vi "InGen.vi"() -> (0 "Variables de planta":u16[](array[numeric]))   [LabVIEW 2017, in "Lib_Esclavo_Ingen.lvlib"]
doc: "Simulador de variables eléctricas. Planta InGEN INC."
uses:
  <vilib>/Analysis/baseanly.llb/Mean (DBL).vi
  Lib_Esclavo_Ingen.lvlib
  <vilib>/Analysis/NI_AALBase.lvlib
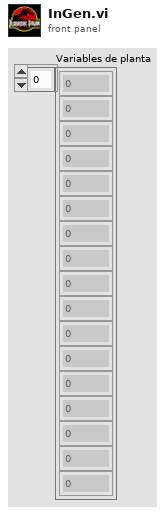
[diagram p1: front panel]
types:
  T1 = enum16{"Tensiones", "Corrientes", "Potencias", "Factores de Potencia", "Frecuencia"}
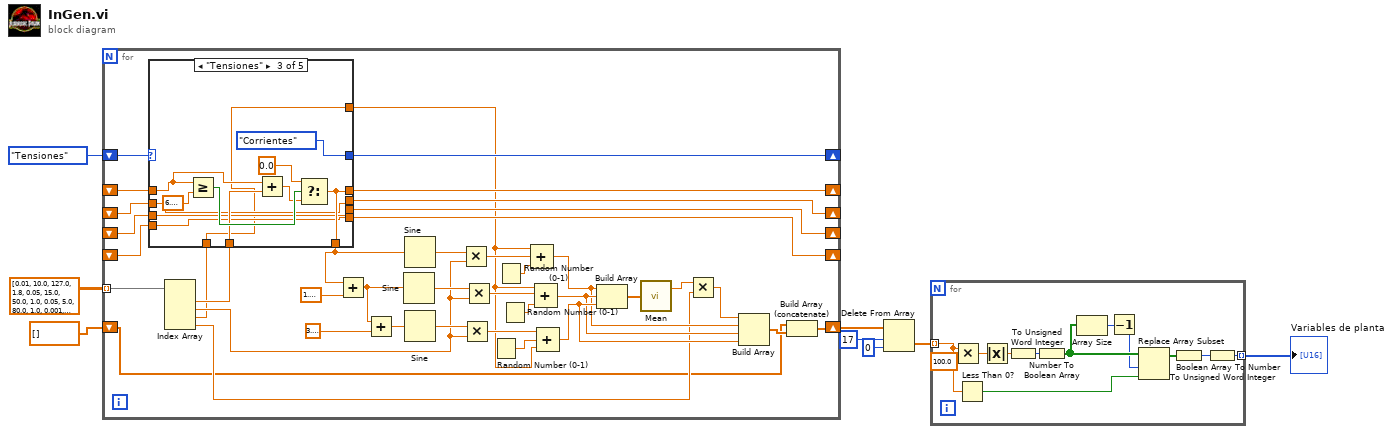
[diagram p0: block diagram]
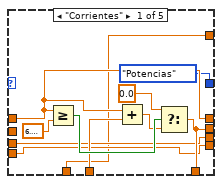
[diagram p2: hidden frame]
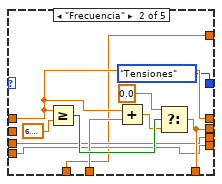
[diagram p3: hidden frame]
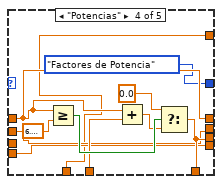
[diagram p4: hidden frame]
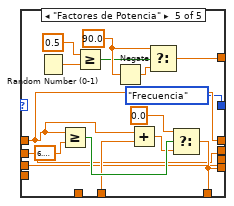
[diagram p5: hidden frame]
diagram:
  n1 = for {
    shift-right: [w13] -> _
    shift-left: T1."Tensiones" -> [w21]
    shift-right: [w28] -> _
    shift-left: _ -> [w27]
    tunnel: dbl[][] [[0.01, 10.0, 127.0, 1.8], [0.05, 15.0, 50.0, 1.0], [0.05, 5.0, 80.0, 1.0], [0.001, 0.5, 90.0, 1.0], [0.001, 0.5, 60.0, 1.0]] -> [w25] mode=indexing
    shift-right: [w17] -> _
    shift-left: _ -> [w20]
    shift-right: [w16] -> _
    shift-left: _ -> [w19]
    shift-right: [w15] -> _
    shift-left: _ -> [w18]
    shift-right: [w9] -> w6
    shift-left: dbl[] [] -> [w10]
    n2 = Index Array(array=w25) -> (element #1=w24:dbl, element #2=w23:dbl, element #3=w12:dbl, element #4=w22:dbl)  [unwired: 4 in]
    n3 = case shown="\"Tensiones\"" w21 {
      tunnel: [w54 w65 w75 w88 w104] -> w28
      tunnel: w27 -> [w54 w65 w77 w88 w104]
      tunnel: w24 -> [w53 w64 w76 w87 w103]
      tunnel: w20 -> [_ _ w74 w85 w101]
      tunnel: w19 -> [w51 w62 w73 _ w100]
      tunnel: w18 -> [w50 w61 w72 w84 _]
      tunnel: [w52 w63 w74 w85 w101] -> w17
      tunnel: [w51 w62 w73 w86 w100] -> w16
      tunnel: [w50 w61 w72 w84 w102] -> w15
      tunnel: [w52 w63 w75 w86 w102] -> w14
      tunnel: [T1."Potencias" T1."Tensiones" T1."Corrientes" T1."Factores de Potencia" T1."Frecuencia"] -> w13
      tunnel: w12 -> [w48 w59 w70 w82 _]
      tunnel: [w48 w59 w70 w82 w93] -> w11
      frame "Corrientes" {
        n4 = Greater Or Equal?(x=w54, y=6.283185307179586) -> (x >= y?=w58:bool)
        n5 = Add(x=w54, y=w53) -> (x+y=w57:dbl)
        n6 = Select(t=0.0, s=w58, f=w57) -> (s? t:f=w52:dbl)
      }
      frame "Frecuencia" {
        n7 = Greater Or Equal?(x=w65, y=6.283185307179586) -> (x >= y?=w69:bool)
        n8 = Add(x=w65, y=w64) -> (x+y=w68:dbl)
        n9 = Select(t=0.0, s=w69, f=w68) -> (s? t:f=w63:dbl)
      }
      frame "Tensiones" {
        n10 = Greater Or Equal?(x=w77, y=6.283185307179586) -> (x >= y?=w81:bool)
        n11 = Add(x=w77, y=w76) -> (x+y=w80:dbl)
        n12 = Select(t=0.0, s=w81, f=w80) -> (s? t:f=w75:dbl)
      }
      frame "Potencias" {
        n13 = Greater Or Equal?(x=w88, y=6.283185307179586) -> (x >= y?=w92:bool)
        n14 = Add(x=w88, y=w87) -> (x+y=w91:dbl)
        n15 = Select(t=0.0, s=w92, f=w91) -> (s? t:f=w86:dbl)
      }
      frame "Factores de Potencia" {
        w97 = 90.0 ("t")
        n16 = Random Number (0-1)() -> (number: 0 to 1=w94:dbl)
        n17 = Greater Or Equal?(x=w104, y=6.283185307179586) -> (x >= y?=w108:bool)
        n18 = Greater Or Equal?(x=0.5, y=w94) -> (x >= y?=w96:bool)
        n19 = Negate(x=w97) -> (-x=w98:dbl)
        n20 = Add(x=w104, y=w103) -> (x+y=w107:dbl)
        n21 = Select(t=w97, s=w96, f=w98) -> (s? t:f=w93:dbl)
        n22 = Select(t=0.0, s=w108, f=w107) -> (s? t:f=w102:dbl)
      }
    }
    n23 = Add(x=w14, y=1.5707963267948966) -> (x+y=w30:dbl)
    n24 = Add(x=w30, y=3.141592653589793) -> (x+y=w32:dbl)
    n25 = Sine(x=w30) -> (sin(x)=w34:dbl)
    n26 = Sine(x=w14) -> (sin(x)=w35:dbl)
    n27 = Sine(x=w32) -> (sin(x)=w33:dbl)
    n28 = Multiply(x=w35, y=w23) -> (x*y=w39:dbl)
    n29 = Multiply(x=w33, y=w23) -> (x*y=w41:dbl)
    n30 = Multiply(x=w34, y=w23) -> (x*y=w40:dbl)
    n31 = Random Number (0-1)() -> (number: 0 to 1=w38:dbl)
    n32 = Random Number (0-1)() -> (number: 0 to 1=w36:dbl)
    n33 = Random Number (0-1)() -> (number: 0 to 1=w37:dbl)
    n34 = Compound Arithmetic op=ADD(w11, w39, w36) -> (w45:dbl)
    n35 = Compound Arithmetic op=ADD(w11, w40, w37) -> (w46:dbl)
    n36 = Compound Arithmetic op=ADD(w41, w38, w11) -> (w47:dbl)
    n37 = Build Array(w45, w46, w47) -> (w42:dbl[])
    n38 = call-poly <vilib>:"Mean.vi"("X"=w42) -> ("mean"=w43:dbl)  [unwired: 1 out]
    n39 = Multiply(x=w43, y=w22) -> (x*y=w44:dbl)
    n40 = Build Array(w44, w45, w46, w47) -> (w26:dbl[])
    n41 = Build Array (concatenate)(w10, w26) -> (w9:dbl[])
  }
  n42 = Delete From Array(array=w6, length=17, index=0) -> (deleted portion=w3:dbl[])  [unwired: 1 out]
  n43 = for {
    tunnel: w3 -> [w117] mode=indexing
    tunnel: [w113] -> w2 mode=indexing
    n44 = Multiply(x=w117, y=100.0) -> (x*y=w119:dbl)
    n45 = Less Than 0?(x=w117) -> (x < 0?=w116:bool)
    n46 = Absolute Value(x=w119) -> (abs(x)=w109:dbl)
    n47 = To Unsigned Word Integer(number=w109) -> (unsigned 16bit integer=w118:u16)
    n48 = Number To Boolean Array(number=w118) -> (Boolean array=w115:bool[])
    n49 = Array Size(array=w115) -> (size(s)=w112:i32)
    n50 = Decrement(x=w112) -> (x-1=w111:i32)
    n51 = Replace Array Subset(array=w115, new element=w116, index=w111) -> (w110:bool[])
    n52 = Boolean Array To Number(Boolean array=w110) -> (number=w114:u32)
    n53 = To Unsigned Word Integer(number=w114) -> (unsigned 16bit integer=w113:u16)
  }
  "Variables de planta" <- w2
